vi "test_Write FXP Register Value.vi"(8 "error in (no error)":errorcluster, 11 "TestCase in":refnum<class "FPGA Register IO Tests.lvclass">) -> (0 "error out":errorcluster, 3 "TestCase out":refnum<class "FPGA Register IO Tests.lvclass">)   [LabVIEW 2020, in "FPGA Register IO Tests.lvclass"]
uses:
  FPGA Register IO Tests.lvclass
  APIs/FPGA Register IO/TypeDefs/FXP Configuration.ctl
  <vilib>/fxp/LVFixedPointRepBitsTypeDef.ctl
  <vilib>/fxp/LVFixedPointRepRangeTypeDef.ctl
  FPGA Register IO Tests.lvclass/FPGA Register IO Tests.ctl
  APIs/FPGA Register IO/Write Methods/Write Data Register/Instances/Write FXP.vi
  APIs/FPGA Register IO/Read Methods/Read Data Register/Instances/Read FXP.vi
  APIs/FPGA Register IO/Write Methods/Write Data Register/Instances/Write U16.vi
  APIs/FPGA Register IO/Write Methods/Write Data Register/Instances/Write U32.vi
  APIs/FPGA Register IO/Write Methods/Write Data Register/Instances/Write U64.vi
  APIs/FPGA Register IO/Write Methods/Write Data Register/Instances/Write U8.vi
  APIs/FPGA Register IO/SubVIs/DBL to FXP Raw.vi
  APIs/FPGA Register IO/SubVIs/FXP Raw to DBL.vi
  APIs/FPGA Register IO/Read Methods/Read Data Register/Instances/Read U16.vi
  APIs/FPGA Register IO/Read Methods/Read Data Register/Instances/Read U32.vi
  APIs/FPGA Register IO/Read Methods/Read Data Register/Instances/Read U64.vi
  APIs/FPGA Register IO/Read Methods/Read Data Register/Instances/Read U8.vi
  APIs/FPGA Register IO/Utilities/Find Register Offset.vi
  APIs/FPGA Register IO/SubVIs/Check Register Data Store.vi
  APIs/FPGA Register IO/Error Handling/Error 6001.vi
  APIs/FPGA Register IO/Error Handling/Error 6000.vi
  APIs/FPGA Register IO/Error Handling/Error 6002.vi
  APIs/FPGA Register IO/Error Handling/Error 6006.vi
  APIs/FPGA Register IO/Error Handling/Error 6003.vi
  <vilib>/FPGAPlugInAG/Dynamic/niLvFpga_Close_Dynamic.vi
  <vilib>/rvi/interface/nirviCloseFPGA/nirviCloseFPGA.xnode
  <vilib>/addons/_JKI Toolkits/VI Tester/TestCase.llb/TestCase.lvclass
  APIs/FPGA Register IO/FPGA Register IO.lvlib
  C:/Program Files (x86)/National Instruments/LabVIEW 2020/vi.lib/addons/_JKI Toolkits/VI Tester/TestCase.llb/TestCase.lvclass
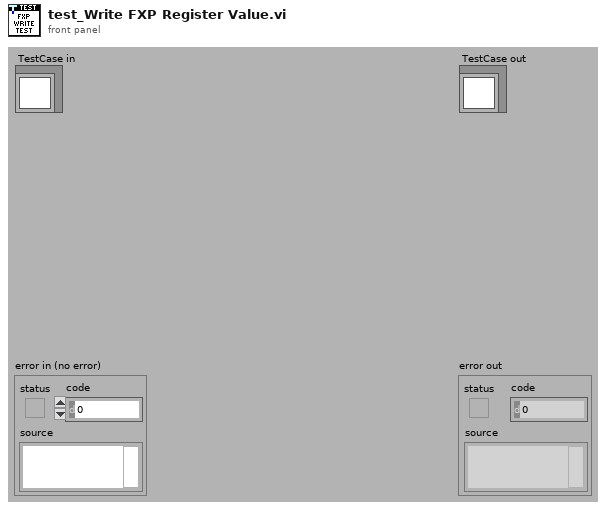
[diagram p1: front panel]
types:
  T1 = typedef "FPGA Register IO.lvlib/FXP Configuration.ctl" = cluster{"FXP Representation":T2, "FXP Range":T3}
  T2 = typedef "LVFixedPointRepBitsTypeDef.ctl" = cluster{"Signed":bool, "Word Length":u32, "Integer Word Length":i32}
  T3 = typedef "LVFixedPointRepRangeTypeDef.ctl" = cluster{"Range Min":dbl, "Range Max":dbl, "Delta":dbl}
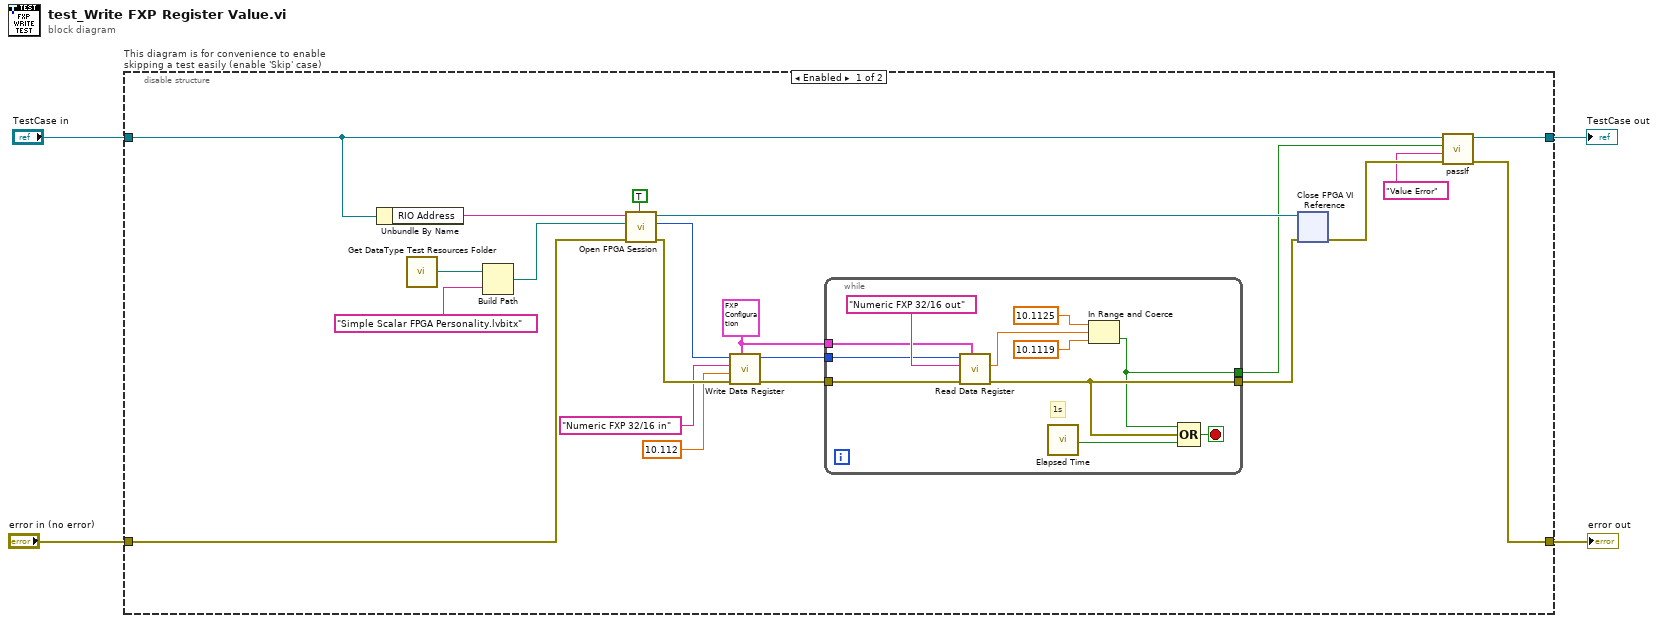
[diagram p0: block diagram]
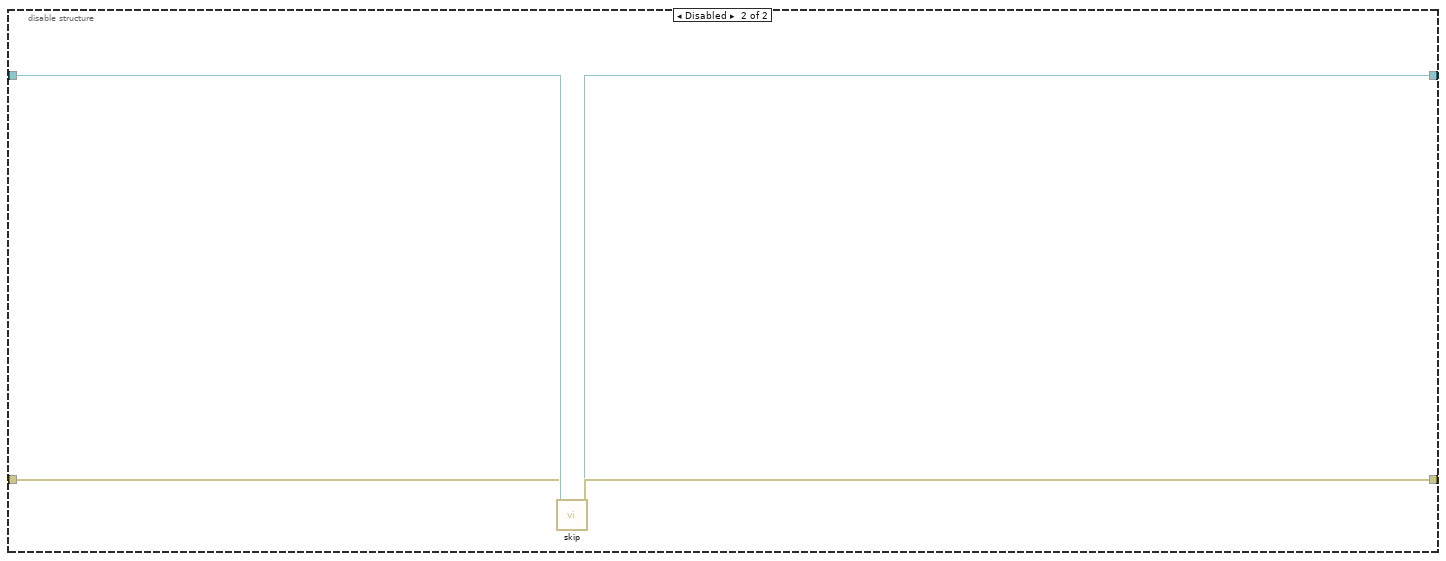
[diagram p2: hidden frame]
diagram:
  n1 = disable-structure "This diagram is for convenience to enable skipping a test easily (enable 'Skip' case)" shown="Enabled" {
    disable-tunnel: "TestCase in" -> [w20 w40]
    disable-tunnel: [w16 w38] -> w1
    disable-tunnel: [w15 w39] -> w3
    disable-tunnel: "error in (no error)" -> [w21 w37]
    frame Enabled {
      w7 = T1 {"FXP Representation"={"Signed"=TRUE, "Word Length"=32, "Integer Word Length"=16}, "FXP Range"={"Range Min"=0.0, "Range Max"=0.0, "Delta"=1.52588e-05}} ("FXP Configuration")
      n2 = Unbundle By Name(w20) -> ("RIO Address"=w14:string)
      n3 = call "Get DataType Test Resources Folder.vi"() -> ("path"=w18:path)
      n4 = Build Path(base path=w18, name or relative path="Simple Scalar FPGA Personality.lvbitx") -> (appended path=w22:path)
      n5 = call "Open FPGA Session.vi"("run when loaded (T)"=TRUE ("Run When Loaded (T)"), "error in"=w21, "bitfile path"=w22, "device address"=w14) -> ("error out"=w13:errorcluster, "session out"=w11:u32, "bitfile reference out"=w24:refnum<k20>)  [unwired: 5 in]
      n6 = call-poly "Write Data Register.vi"("FXP Configuration"=w7, "error in"=w13, "DBL Value"=10.112 ("value in"), "register name"="Numeric FXP 32/16 in", "session in"=w11) -> ("error out"=w9:errorcluster, "session out"=w10:u32)  [unwired: 5 in]
      n7 = while {
        tunnel: [w32] -> w5
        tunnel: w9 -> [w35]
        tunnel: w10 -> [w34]
        tunnel: [w29] -> w6
        tunnel: w7 -> [w30]
        stop <- w33 stop-if-true
        # "1s"
        n8 = call-poly "Read Data Register.vi"("FXP Configuration"=w30, "error in"=w35, "register name"="Numeric FXP 32/16 out" ("registerName"), "session in"=w34) -> ("error out"=w32:errorcluster, "DBL Value"=w26:dbl)  [unwired: 5 in, 1 out]
        n9 = call "Elapsed Time"() -> ("Time has Elapsed"=w31:bool)  [unwired: 12 in, 7 out]
        n10 = In Range and Coerce(upper limit=10.1125 ("DBL Value"), x=w26, lower limit=10.1119 ("DBL Value")) -> (In Range?=w29:bool)  [unwired: 1 out]
        n11 = Compound Arithmetic op=OR(w29, w32, w31) -> (w33:bool)
      }
      n12 = xnode "Close FPGA VI Reference"("FPGA VI Reference In"=w24, "error in"=w5) -> ("error out"=w19:errorcluster)
      n13 = call-dynamic "passIf.vi"("error in (no error)"=w19, "message (\"\")"="Value Error" ("message (\"\")"), "pass"=w6, "TestCase in"=w20) -> ("error out"=w15:errorcluster, "TestCase out"=w16:refnum<class "FPGA Register IO Tests.lvclass">)  [unwired: 6 in]
    }
    frame Disabled {
      # "skip test result while test is under development"
      n14 = call <vilib>:"skip.vi"("error in (no error)"=w37, "TestCase in"=w40) -> ("error out"=w39:errorcluster, "TestCase out"=w38:refnum<class "FPGA Register IO Tests.lvclass">)  [unwired: 8 in]
    }
  }
  "error out" <- w3
  "TestCase out" <- w1
